vi "Generate Sine Wave for Digital Audio - Crosstalk.vi"(5 "interferrer channel":i32, 7 "number of channels":i32, 9 "phase":dbl, 10 "gain":dbl=0.5, 11 "frequency":dbl=0.5) -> (3 "Signal Properties":T1)   [LabVIEW 2021, in "Crosstalk_Audio DAC.lvlib"]
uses:
  <vilib>/PDM Acquisition Toolkit/host/Classes/Tasks/I2S Output/Control/SignalProperties.ctl
  <vilib>/PDM Acquisition Toolkit/host/Classes/Channels/I2S Ouput/Controls/GenerationChannelProperties.ctl
  Crosstalk_Audio DAC.lvlib
  <vilib>/Analysis/NI_AALBase.lvlib
  <vilib>/PDM Acquisition Toolkit/host/Classes/Channels/I2S Ouput/I2S Output Channel.lvclass
  <vilib>/PDM Acquisition Toolkit/host/Classes/Tasks/I2S Output/I2S Output Task.lvclass
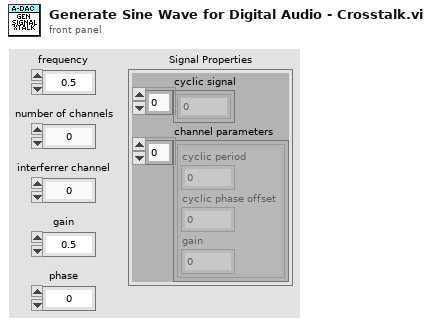
[diagram p1: front panel]
types:
  T1 = typedef "PDM Acquisition Class Library.lvlib/I2S Output Task.lvclass/SignalProperties.ctl" = cluster{"cyclic signal":dbl[], "channel parameters":T2[]}
  T2 = typedef "PDM Acquisition Class Library.lvlib/I2S Output Channel.lvclass/GenerationChannelProperties.ctl" = cluster{"cyclic period":dbl, "cyclic phase offset":dbl, "gain":dbl}
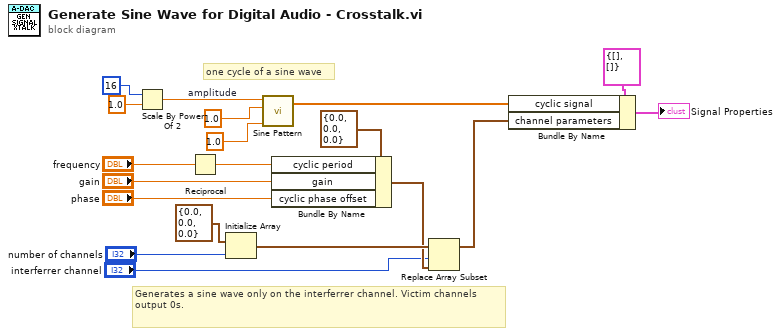
[diagram p0: block diagram]
diagram:
  w19 = 1.0  # amplitude
  # "one cycle of a sine wave"
  # "Generates a sine wave only on the interferrer channel. Victim channels output 0s."
  n1 = Scale By Power Of 2(n=i16 16, x=1.0) -> (x*2^n=w11:dbl)
  n2 = Reciprocal(x="frequency") -> (1/x=w8:dbl)
  n3 = Initialize Array(T2 {"cyclic period"=0.0, "cyclic phase offset"=0.0, "gain"=0.0}, "number of channels") -> (w4:T2[])
  n4 = call <vilib>:"Sine Pattern.vi"("cycles"=1.0, "amplitude"=w19, "samples"=w11) -> ("Sinusoidal Pattern"=w13:dbl[])  [unwired: 1 in, 1 out]
  n5 = Bundle By Name(cluster=T2 {"cyclic period"=0.0, "cyclic phase offset"=0.0, "gain"=0.0}, "cyclic period"=w8, "gain"="gain", "cyclic phase offset"="phase") -> (w3:T2)
  n6 = Replace Array Subset(array=w4, new element=w3, index="interferrer channel") -> (w1:T2[])
  n7 = Bundle By Name(cluster=T1 {"cyclic signal"=[], "channel parameters"=[]} ("Signal Properties"), "cyclic signal"=w13, "channel parameters"=w1) -> (→"Signal Properties":T1)
